vi "PH_BL-Master.PC Remote Controlled.vi"(0 "i ref in":refnum<vi>, 2 "Remote controlled":bool, 5 "error in (no error)":errorcluster) -> (14 "i ref out":refnum<vi>, 19 "error out":errorcluster)   [LabVIEW 2014, in "PH_BL-Master.lvlib"]
doc: "This VI enables or disables GUI elements."
uses:
  PH_BL-Master.lvlib
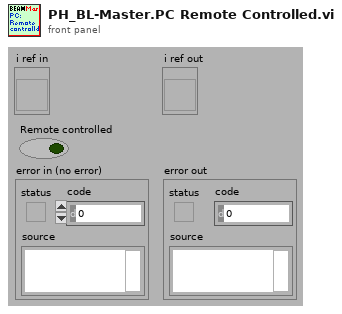
[diagram p1: front panel]
types:
  T1 = typedef "PH_BL-Master.lvlib/PH_BL-Master.i attribute.ctl" = cluster{"Remote controlled":bool, "Boolean Condition Service Subscriber":refnum<vi>[], "Picture Condition Service Subscriber":refnum<vi>[], "R2S":cluster{"GUI Ref":refnum<vi>, "State":bool}, "Vacua":cluster{"GUI Ref":refnum<vi>, "Limit":dbl, "Curr Value":dbl, "in range":bool}[], "O2 Inspection":cluster{"GUI Ref":refnum<vi>, "Concentration":dbl, "State":T2}[], "Boolean Status Service Subscriber":cluster{"GUI Ref":refnum<vi>, "Status":T2, "no Link?":bool, "Status Subscriber Class":T3}[], "Picture Status Service Subscriber":cluster{"GUI Ref":refnum<vi>, "Status":T2, "no Link?":bool, "Status Subscriber Class":T3}[], "6P 4Q Service Subscriber":cluster{"GUI Ref":refnum<vi>, "Selector":T4, "no Link?":bool}[], "Index of latest 6P 4Q changing Instance":i32, "Index of latest Picture Status changing Instance":i32, "Index of latest Boolean Status changing Instance":i32, "Vision ID on same Node":string, "Start Phase over?":bool, "GUI Ref Delete":refnum<vi>}
  T2 = typedef "PH_StatusHandler.lvlib/PH_StatusHandler.Status.ctl" = i16
  T3 = typedef "PH_BL-Master.lvlib/PH_BL-Master.Status Subscriber Class.ctl" = enum16{"unknown", "Switch", "BB", "6P Switch", "Switch GUI", "Switch and 6P State", "Force Sensor"}
  T4 = typedef "PH_4_Pos_Selector.lvlib/PH_4_Pos_Selector.Position Selector.ctl" = u16
  T5 = enum8{"Enabled", "Disabled", "Disabled and Grayed Out"}
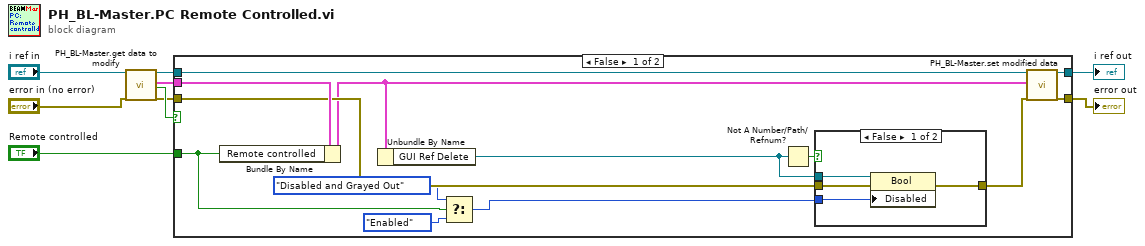
[diagram p0: block diagram]
diagram:
  n1 = call "PH_BL-Master.get data to modify.vi"("i ref in"="i ref in", "error in (no error)"="error in (no error)") -> ("i ref out"=w3:refnum<vi>, "i attribute"=w7:T1, "timed out"=w8:bool, "error out"=w5:errorcluster)  [unwired: 14 in]
  n2 = case shown="False" w8 {
    tunnel: w3 -> [w22 w29]
    tunnel: [w21 w29] -> w4
    tunnel: w5 -> [w18 w28]
    tunnel: [w20 w28] -> w6
    tunnel: w7 -> [w19 _]
    tunnel: "Remote controlled" -> [w10 _]
    frame False {
      n3 = Bundle By Name(cluster=w19, "Remote controlled"=w10) -> (w16:T1)
      n4 = Unbundle By Name(w16) -> ("GUI Ref Delete"=w15:refnum<vi>)
      n5 = Select(t=T5."Disabled and Grayed Out" ("Disabled"), s=w10, f=T5."Enabled" ("Disabled")) -> (s? t:f=w12:T5)
      n6 = Not A Number/Path/Refnum?(number/path/refnum=w15) -> (NaN/Path/Refnum?=w14:bool)
      n7 = case shown="False" w14 {
        tunnel: w18 -> [w26 w27]
        tunnel: [w25 w27] -> w17
        tunnel: w15 -> [w24 _]
        tunnel: w12 -> [w23 _]
        frame False {
          n8 = property class="Bool"(reference=w24, error in=w26, "Disabled"=w23) -> (error out=w25:errorcluster)  [unwired: 1 out]
        }
        frame True {
        }
      }
      n9 = call "PH_BL-Master.set modified data.vi"("i ref in"=w22, "i attribute"=w16, "error in (no error)"=w17) -> ("i ref out"=w21:refnum<vi>, "error out"=w20:errorcluster)  [unwired: 15 in]
    }
    frame True {
    }
  }
  "error out" <- w6
  "i ref out" <- w4
